vi "AB_API Attribute Error_Path.vi"(8 "error in (no error)":errorcluster, 11 "path":path) -> (0 "error out":errorcluster)   [LabVIEW 2020]
uses:
  <resource>/Framework/Providers/Common/provcom_StringGlobals.vi
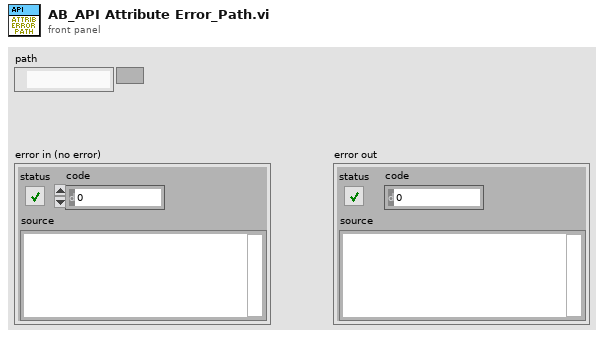
[diagram p1: front panel]
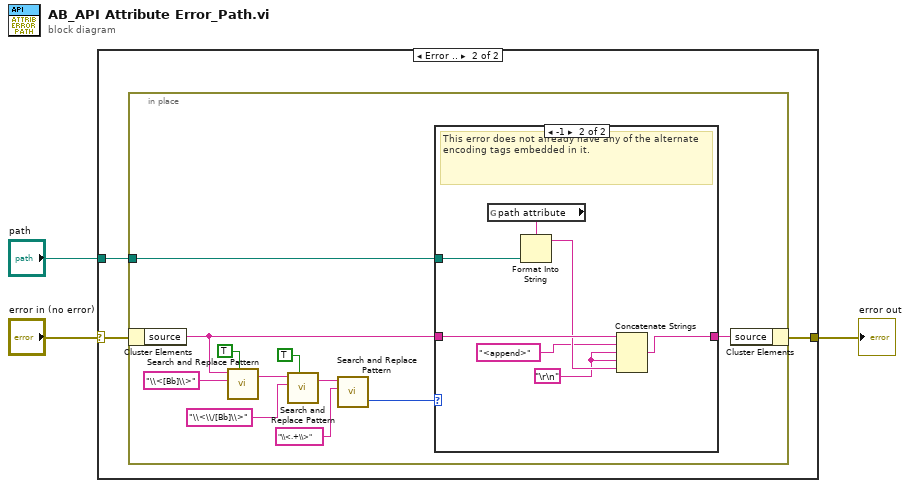
[diagram p0: block diagram]
diagram:
  n1 = case shown="Error .." "error in (no error)" {
    selector: "error in (no error)" -> [w4 w6]
    tunnel: "path" -> [_ w7]
    tunnel: [w4 w5] -> w1
    frame No Error {
    }
    frame Error {
      n2 = in-place {
        in-place-border: w7 -> [w18]
        n3 = in-place-cluster #1(w6) -> ("source"=w16:string)
        n4 = call <vilib>:"Search and Replace Pattern.vi"("string"=w16, "regular expression (\"\")"="\\<[Bb]\\>" ("regular expression (\"\")"), "replace all? (F)"=TRUE) -> ("result string"=w11:string)  [unwired: 2 in, 1 out]
        n5 = call <vilib>:"Search and Replace Pattern.vi"("string"=w11, "regular expression (\"\")"="\\<\\/[Bb]\\>" ("regular expression (\"\")"), "replace all? (F)"=TRUE) -> ("result string"=w10:string)  [unwired: 2 in, 1 out]
        n6 = call <vilib>:"Search and Replace Pattern.vi"("string"=w10, "regular expression (\"\")"="\\<.+\\>" ("regular expression (\"\")")) -> ("offset past match"=w8:i32)  [unwired: 3 in, 1 out]
        n7 = case shown="-1" w8 {
          tunnel: w18 -> [_ w26]
          tunnel: w16 -> [w19 w25]
          tunnel: [w19 w24] -> w15
          frame Default {
          }
          frame -1 {
            w21 = "\r\n"
            # "This error does not already have any of the alternate encoding tags embedded in it."
            n8 = global read "provcom_StringGlobals.vi" "path attribute"() -> (w23:string)
            n9 = Format Into String(format string=w23, w26) -> (resulting string=w22:string)  [unwired: 2 in, 1 out]
            n10 = Concatenate Strings(w25, "<append>" ("string"), w21, w21, w22) -> (w24:string)
          }
        }
        n11 = in-place-cluster #1("source"=w15) -> (w5:errorcluster)
      }
    }
  }
  "error out" <- w1
